vi "Log Data.vi"(0 "Test Inputs":T2={"Load Current in A"=0.0, "Frequency in Hz"=[], "Input Voltage in V"=0.0, "FGen Peak-Peak Voltage in V"=0.0, "Resolution bandwidth in %"=20000000.0, "Sampling Rate multiplier"=1000.0, "Take PSRR snapshot?"=FALSE, "Acquisition Time(s)"=0.0, "Horizontal Timing"=enum."Calculate Sampling Rate", "Advance Setting"={"Prepare"={"Load SMU Output Function"=enum."VoltageSource"}, "Stimulus and Measure"={"Loop Delay"=0, "Autoset Sampling Rate?"=TRUE, "Search Tolerance (+/- % of Freq.)"=0.0}}} {"Input Voltage in V" format="%#.5g"; "Load Current in A" format="%#.5g"}, 5 "Test Results":T1 {"Record Length in S" format="%#.5g"; "Sample Rate in S/s" format="%#.5g"; "PSRR in dB" format="%#.5g"; "Frequency in Hz" format="%#.5g"; "Detected Vin_ac_pp in V" format="%#.5g"; "Detected Vout_ac_pp in V" format="%#.5g"}, 7 "DataLogger File Path":path, 11 "error in (no error)":errorcluster) -> (15 "error out":errorcluster)   [LabVIEW 2020, in "LDO PSRR.lvlib"]
uses:
  LDO PSRR.lvlib
  Typedefs/Test Inputs.ctl
  Typedefs/Advance Test Input.ctl
  Reusables/Instrument APIs/Load Output Function.ctl
  Typedefs/Test Results.ctl
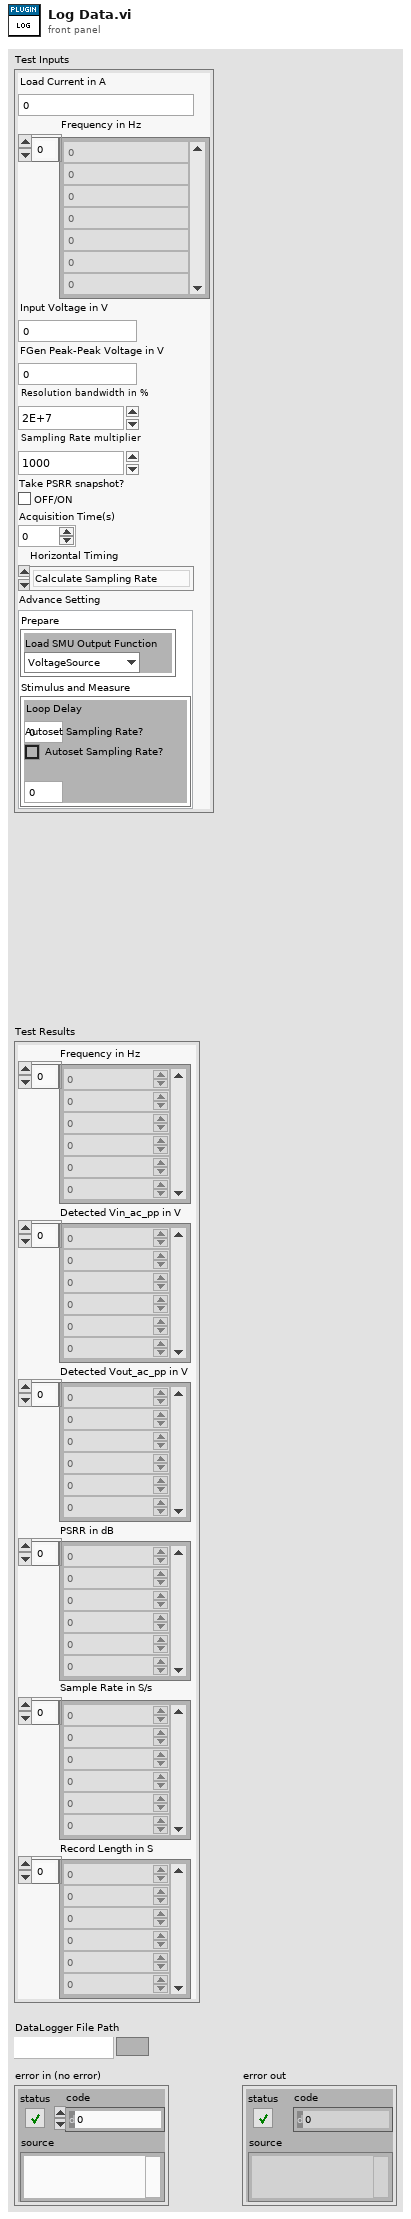
[diagram p1: front panel]
types:
  T1 = typedef "LDO PSRR.lvlib/Test Results.ctl" = cluster{"Frequency in Hz":dbl[], "Detected Vin_ac_pp in V":dbl[], "Detected Vout_ac_pp in V":dbl[], "PSRR in dB":dbl[], "Sample Rate in S/s":dbl[], "Record Length in S":dbl[]}
  T2 = typedef "LDO PSRR.lvlib/Test Inputs.ctl" = cluster{"Load Current in A":dbl, "Frequency in Hz":dbl[], "Input Voltage in V":dbl, "FGen Peak-Peak Voltage in V":dbl, "Resolution bandwidth in %":dbl, "Sampling Rate multiplier":dbl, "Take PSRR snapshot?":bool, "Acquisition Time(s)":dbl, "Horizontal Timing":enum32{"Calculate Sampling Rate", "Calculate Acquisition Time", "Calculate Record Length"}, "Advance Setting":T3}
  T3 = typedef "LDO PSRR.lvlib/Advance Test Input.ctl" = cluster{"Prepare":cluster{"Load SMU Output Function":T4}, "Stimulus and Measure":cluster{"Loop Delay":u32, "Autoset Sampling Rate?":bool, "Search Tolerance (+/- % of Freq.)":dbl}}
  T4 = typedef "Load Output Function.ctl" = enum16{"VoltageSource", "CurrentSource"}
  T5 = enum16{"open", "replace", "create", "open or create", "replace or create", "replace or create with confirmation"}
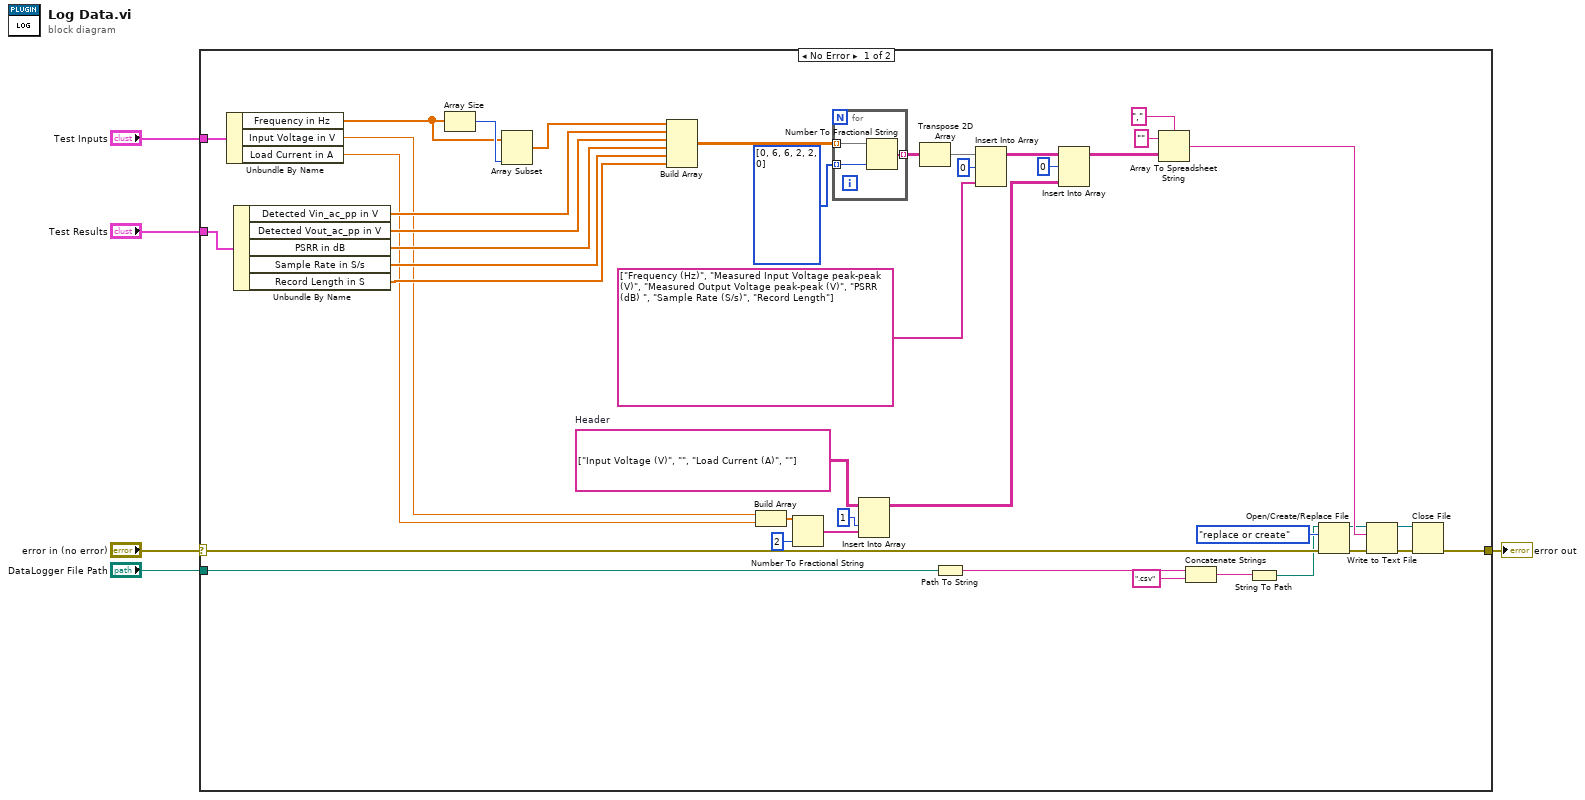
[diagram p0: block diagram]
diagram:
  n1 = case shown="No Error" "error in (no error)" {
    selector: "error in (no error)" -> [w34 w51]
    tunnel: [w39 w51] -> w4
    tunnel: "Test Inputs" -> [w47 _]
    tunnel: "Test Results" -> [w46 _]
    tunnel: "DataLogger File Path" -> [w33 _]
    frame No Error {
      w15 = string[][] [["Input Voltage (V)", ""], ["Load Current (A)", ""]]  # Header
      n2 = Unbundle By Name(w47) -> ("Frequency in Hz"=w31:dbl[], "Input Voltage in V"=w8:dbl, "Load Current in A"=w7:dbl)
      n3 = Unbundle By Name(w46) -> ("Detected Vin_ac_pp in V"=w43:dbl[], "Detected Vout_ac_pp in V"=w44:dbl[], "PSRR in dB"=w45:dbl[], "Sample Rate in S/s"=w30:dbl[], "Record Length in S"=w29:dbl[])
      n4 = Array Size(array=w31) -> (size(s)=w32:i32)
      n5 = Array Subset(array=w31, length=w32) -> (w35:dbl[])  [unwired: 1 in]
      n6 = Build Array(w35, w43, w44, w45, w30, w29) -> (w42:dbl[][])
      n7 = Build Array(w8, w7) -> (w16:dbl[])
      n8 = Number To Fractional String(number=w16, precision (6)=i16 2) -> (F-format string=w14:string[])  [unwired: 2 in]
      n9 = for {
        tunnel: w42 -> [w50] mode=indexing
        tunnel: [w49] -> w28 mode=indexing
        tunnel: i16[] [0, 6, 6, 2, 2, 0] ("precision (6)") -> [w48] mode=indexing
        n10 = Number To Fractional String(number=w50, precision (6)=w48) -> (F-format string=w49:string[])  [unwired: 2 in]
      }
      n11 = Insert Into Array(array=w15, index (col)=1 ("index (row)"), new element=w14) -> (w9:string[][])  [unwired: 1 in]
      n12 = Transpose 2D Array(2D array=w28) -> (transposed array=w27:string[][])
      n13 = Path To String(path=w33) -> (string=w18:string)
      n14 = Insert Into Array(array=w27, index (row)=0, new element=string[] ["Frequency (Hz)", "Measured Input Voltage peak-peak (V)", "Measured Output Voltage peak-peak (V)", "PSRR (dB) ", "Sample Rate (S/s)", "Record Length"] ("new element/subarray")) -> (w11:string[][])  [unwired: 1 in]
      n15 = Insert Into Array(array=w11, index (row)=0, new element=w9) -> (w10:string[][])  [unwired: 1 in]
      n16 = Array To Spreadsheet String(delimiter (Tab)=",", array=w10, 3:"" ("format string")) -> (spreadsheet string=w36:string)
      n17 = Concatenate Strings(w18, ".csv" ("format string")) -> (w19:string)
      n18 = String To Path(string=w19) -> (path=w17:path)
      n19 = Open/Create/Replace File(file path (use dialog)=w17, error in=w34, operation (0:open)=T5."replace or create") -> (refnum out=w23:refnum<file>, error out=w25:errorcluster)  [unwired: 3 in, 1 out]
      n20 = Write to Text File(file (use dialog)=w23, text=w36, error in=w25) -> (refnum out=w22:refnum<file>, error out=w24:errorcluster)  [unwired: 1 in, 1 out]
      n21 = Close File(refnum=w22, error in=w24) -> (error out=w39:errorcluster)  [unwired: 1 out]
    }
    frame Error {
    }
  }
  "error out" <- w4
